vi "ZAlign_Delete_Decos.vi"(0 "Panel in":refnum<vi>, 5 "Decor Refnum":refnum<vi>, 11 "error in (no error)":errorcluster) -> (15 "error out":errorcluster)   [LabVIEW 2014, in "ZAlign.lvlib"]
doc: "ZAlign.lvlib:ZAlign_Delete_Decos.vi\n----------------------------------------------\nlöscht nicht benötigte Decos und löst die Gruppierung auf.\n\nInputs:\n---------------------\n- Panel in : Refnum; \n- Decor Refnum : Refnum; \n- error in (no error) : Cluster; \n\nOutputs:\n---------------------\n- error out : Cluster; \n\n----------------------------------------------\n17.03.2015 jcm\nZühlke Engineering AG\nCH-8952 Schlieren\nwww.zuehlke.com"
uses:
  ZAlign.lvlib
panel:
  # "Connector Pane"
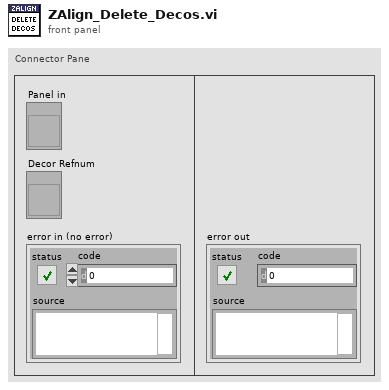
[diagram p1: front panel]
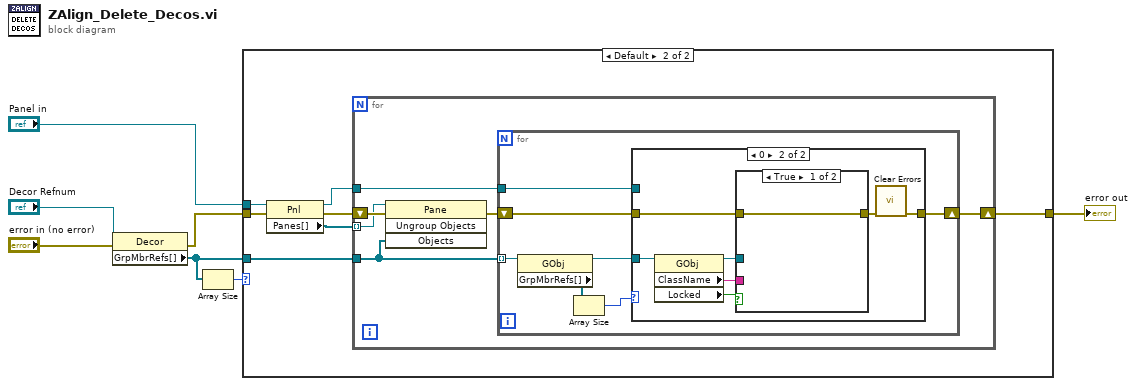
[diagram p0: block diagram]
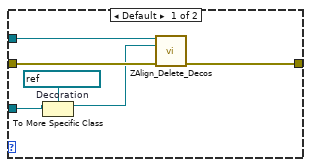
[diagram p3: hidden frame]
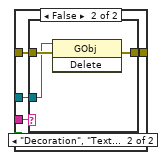
[diagram p4: hidden frame]
diagram:
  n1 = property class="Decor"(reference="Decor Refnum", error in="error in (no error)") -> (error out=w2:errorcluster, "GrpMbrRefs[]"=w6:refnum<vi>[])  [unwired: 1 out]
  n2 = Array Size(array=w6) -> (size(s)=w7:i32)
  n3 = case shown="Default" w7 {
    tunnel: [w8 w15] -> w1
    tunnel: w2 -> [w8 w13]
    tunnel: w6 -> [_ w12]
    tunnel: "Panel in" -> [_ w11]
    frame 0 {
    }
    frame Default {
      n4 = property class="Pnl"(reference=w11, error in=w13) -> (reference out=w9:refnum<vi>, error out=w14:errorcluster, "Panes[]"=w10:refnum<vi>[])
      n5 = for {
        tunnel: w12 -> [w19]
        tunnel: w10 -> [w17] mode=indexing
        shift-right: [w21] -> w15
        shift-left: w14 -> [w20]
        tunnel: w9 -> [w16]
        n6 = invoke class="Pane" method="Ungroup Objects"(reference=w17, error in=w20, "Objects"=w19) -> (error out=w18:errorcluster)  [unwired: 1 in, 3 out]
        n7 = for {
          tunnel: w19 -> [w26] mode=indexing
          shift-right: [w28] -> w21
          shift-left: w18 -> [w27]
          tunnel: w16 -> [w22]
          n8 = property class="GObj"(reference=w26) -> (reference out=w25:refnum<vi>, "GrpMbrRefs[]"=w24:refnum<vi>[])  [unwired: 1 in, 1 out]
          n9 = Array Size(array=w24) -> (size(s)=w23:i32)
          n10 = case shown="0" w23 {
            tunnel: [w33 w41] -> w28
            tunnel: w27 -> [w34 w40]
            tunnel: w25 -> [w30 w36]
            tunnel: w22 -> [w32 _]
            frame Default {
              w31 = refnum<vi> refnum  # Decoration
              n11 = To More Specific Class(target class=w31, reference=w30) -> (specific class reference=w29:refnum<vi>)  [unwired: 1 in, 1 out]
              n12 = call "ZAlign_Delete_Decos.vi"("Panel in"=w32, "Decor Refnum"=w29, "error in (no error)"=w34) -> ("error out"=w33:errorcluster)  [unwired: 12 in]
            }
            frame 0 {
              n13 = property class="GObj"(reference=w36) -> (reference out=w38:refnum<vi>, "ClassName"=w37:string, "Locked"=w35:bool)  [unwired: 1 in, 1 out]
              n14 = case shown="True" w35 {
                tunnel: w40 -> [w42 w46]
                tunnel: [w42 w45] -> w39
                tunnel: w38 -> [_ w44]
                tunnel: w37 -> [_ w43]
                frame True {
                }
                frame False {
                  n15 = case shown="\"Decoration\", \"Text\"" w43 {
                    tunnel: w46 -> [w47 w50]
                    tunnel: [w47 w49] -> w45
                    tunnel: w44 -> [_ w48]
                    frame Default {
                    }
                    frame "Decoration", "Text" {
                      n16 = invoke class="GObj" method="Delete"(reference=w48, error in=w50) -> (error out=w49:errorcluster)  [unwired: 1 in, 2 out]
                    }
                  }
                }
              }
              n17 = call <vilib>:"Clear Errors.vi"("error in (no error)"=w39) -> ("error out"=w41:errorcluster)  [unwired: 5 in, 1 out]
            }
          }
        }
      }
    }
  }
  "error out" <- w1
